vi "Nyquist Plot of a Filter.vi"() -> ()   [LabVIEW 2020]
doc: "Computes the frequency response function of a digital filter and displays the attenuation versus the frequency, as well as the imaginary part versus the real part (i.e., Nyquist plot). This example uses a white noise signal as the stimulus of the filter and measures the frequency response between this stimulus and the response of the filter."
uses:
  <vilib>/measure/macond.llb/IIR Filter for 1 Chan.vi
  <vilib>/measure/maspectr.llb/Frequency Response Function (Real-Im) 1-1.vi
  <vilib>/measure/NI_MABase.lvlib
  <vilib>/measure/NI_MAPro.lvlib
panel:
  in  "Filter specifications":T1={"Topology"=enum."Butterworth", "Type"=enum."Bandpass", "Order"=3, "Lower Fc"=1000.0, "Upper Fc"=2000.0, "PB Ripple"=0.025, "SB Attenuation"=90.0} {"SB Attenuation" format="%#.6g"; "PB Ripple" format="%#.6g"; "Upper Fc" format="%#.6g"; "Lower Fc" format="%#.6g"}
  out "Frequency response":cluster{"f0":dbl, "df":dbl, dbl[]}(graph)
  out "Nyquist plot":T2(graph)
  in  "Stop":bool
  # "Overview: Demonstrates the use of the Frequency Response Function (Real-Im) VI to measure and graph the Nyquist plot of a filter.\nRequirements: LabVIEW Full Development System\nInstructions: \n1. Run the VI.\n2. Move the frequency cursor in the Frequency response graph and see the corresponding location move in the Nyquist plot.\n3. Change the Filter specifications and watch the Nyquist plot and Frequency response form.\n4. Click Stop to stop the VI."
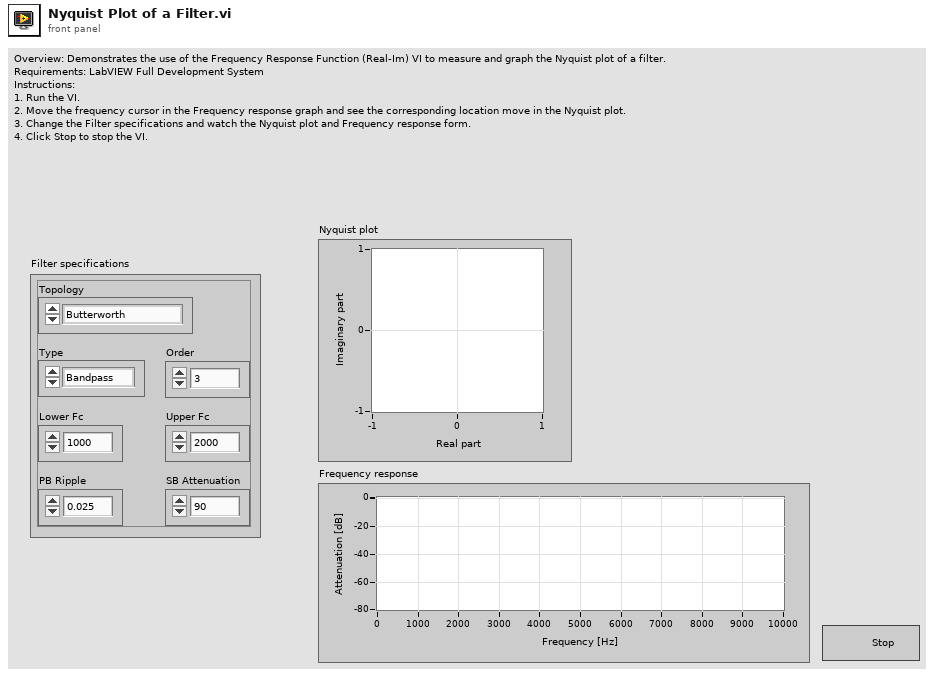
[diagram p1: front panel]
types:
  T1 = cluster{"Topology":enum16{"Off", "Butterworth", "Chebyshev", "Inverse Chebyshev", "Elliptic", "Bessel"}, "Type":enum16{"Lowpass", "Highpass", "Bandpass", "Bandstop"}, "Order":i32, "Lower Fc":dbl, "Upper Fc":dbl, "PB Ripple":dbl, "SB Attenuation":dbl}
  T2 = cluster{"real part":dbl[], "imaginary part":dbl[]}
  T3 = cluster{"averaging mode":enum16{"No averaging", "Vector averaging", "RMS averaging", "Peak hold"}, "weighting mode":enum16{"Linear", "Exponential"}, "number of averages":u32}
  T4 = enum16{"None ", "Hanning", "Hamming", "Blackman-Harris", "Exact Blackman", "Blackman", "Flat Top", "4 Term B-Harris ", "7 Term B-Harris", "Low Sidelobe"}
  T5 = cluster{"f0":dbl, "df":dbl, "imaginary part":dbl[]}
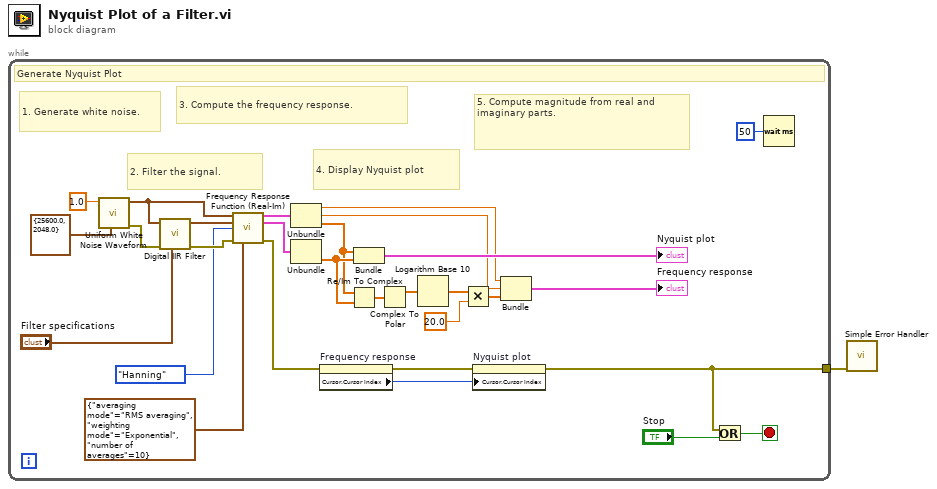
[diagram p0: block diagram]
diagram:
  n1 = while {
    tunnel: [w4] -> w1
    stop <- w5 stop-if-true
    # "5. Compute magnitude from real and imaginary parts."
    # "4. Display Nyquist plot"
    # "2. Filter the signal."
    # "3. Compute the frequency response."
    # "1. Generate white noise."
    # "Generate Nyquist Plot"
    n2 = call <vilib>:"Uniform White Noise Waveform.vi"("sampling info"=cluster{"Fs":dbl, "#s":dbl} {"Fs"=25600.0, "#s"=2048.0}, "amplitude"=1.0) -> ("error out"=w9:errorcluster, "signal out"=w28:waveform(dbl))  [unwired: 8 in]
    n3 = call-poly <vilib>:"Digital IIR Filter.vi"("IIR filter specifications"="Filter specifications", "error in (no error)"=w9, "signal in"=w28) -> ("error out"=w27:errorcluster, "signal out"=w29:waveform(dbl))  [unwired: 6 in, 1 out]
    n4 = call-poly <vilib>:"Frequency Response Function (Real-Im).vi"("time signal X"=w28, "time signal Y"=w29, "window"=T4."Hanning", "error in (no error)"=w27, "averaging parameters"=T3 {"averaging mode"=enum."RMS averaging", "weighting mode"=enum."Exponential", "number of averages"=10}) -> ("real part"=w26:cluster{"f0":dbl, "df":dbl, "real part":dbl[]}, "imaginary part"=w25:T5, "error out"=w7:errorcluster)  [unwired: 5 in, 3 out]
    n5 = Unbundle(w26) -> ("f0"=w18:dbl, "df"=w17:dbl, "real part"=w21:dbl[])
    n6 = Unbundle(w25) -> ("imaginary part"=w22:dbl[])  [unwired: 2 out]
    n7 = property on="Frequency response" class="WFGraph (strict)"(error in=w7) -> (error out=w6:errorcluster, "Cursor.Cursor Index"=w13:i32)  [unwired: 1 in, 1 out]
    n8 = Re/Im To Complex(1:w22, 2:w21) -> (0:w20:cdb[])
    n9 = Bundle("real part"=w21, "imaginary part"=w22) -> (→"Nyquist plot":T2)  [unwired: 1 in]
    n10 = Complex To Polar(r * e^(i*theta)=w20) -> (r=w19:dbl[])  [unwired: 1 out]
    n11 = Logarithm Base 10(1:w19) -> (0:w15:dbl[])
    n12 = Multiply(x=w15, y=20.0) -> (x*y=w14:dbl[])
    n13 = property on="Nyquist plot" class="XYGraph (strict)"(error in=w6, "Cursor.Cursor Index"=w13) -> (error out=w4:errorcluster)  [unwired: 1 in, 1 out]
    n14 = Bundle("f0"=w18, "df"=w17, w14) -> (→"Frequency response":cluster{"f0":dbl, "df":dbl, dbl[]})  [unwired: 1 in]
    n15 = Or(x=w4, y="Stop") -> (x .or. y?=w5:bool)
    n16 = Wait (ms)(milliseconds to wait=u32 50) -> ()  [unwired: 1 out]
  }
  n17 = call <vilib>:"Simple Error Handler.vi"("error in (no error)"=w1) -> ()  [unwired: 4 in, 5 out]
